vi "PH_VacuumControl.PC Write PSDB.vi"(0 "i ref in":refnum<vi>, 5 "error IO":errorcluster) -> (14 "i ref out":refnum<vi>, 19 "error out":errorcluster)   [LabVIEW 2014, in "PH_VacuumControl.lvlib"]
doc: "This is the proc case which writes data to the PHELIX shot data base."
uses:
  PH_VacuumControl.lvlib
  PH_PSDBWriter/PH_PSDBWriter.2D dataset.ctl
  User/Eisenbarth/psdb_lv/PSDB_AxisDescription.ctl
  PH_PSDBWriter/PH_PSDBWriter.Numeric dataset.ctl
  PH_PSDBWriter/PH_PSDBWriter.lvlib
  User/Eisenbarth/psdb_lv/PSDB.lvlib
  PH_Common/PH_Common.lvlib
panel:
  in  "2D data":T1
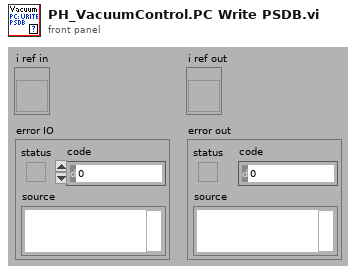
[diagram p1: front panel]
types:
  T1 = typedef "PH_PSDBWriter.lvlib/PH_PSDBWriter.2D dataset.ctl" = cluster{"name":string, "data":dbl[][], "axis description":T2}
  T2 = typedef "PSDB.lvlib/PSDB_AxisDescription.ctl" = cluster{"x axis label":string, "y axis label":string, "x axis unit":string, "y axis unit":string}
  T3 = typedef "PH_PSDBWriter.lvlib/PH_PSDBWriter.Numeric dataset.ctl" = cluster{"name":string, "data":dbl, "unit":string}
  T4 = typedef "PH_VacuumControl.lvlib/PH_VacuumControl.i attribute.ctl" = cluster{"GUI Refs":cluster{"Exit":refnum<vi>, "Set Unit":refnum<vi>, "Device found":refnum<vi>, "Busy":refnum<vi>, "State":refnum<vi>, "Delete":refnum<vi>, "Channels":refnum<vi>, "Channel Name":refnum<vi>, "Trend":refnum<vi>, "Logarithmic":refnum<vi>, "Limit reached":refnum<vi>, "Channel Name 1 MT":refnum<vi>, "Channel Name 2 MT":refnum<vi>, "Trend MT":refnum<vi>, "Logarithmic MT":refnum<vi>, "Limit reached MT":refnum<vi>}, "Device found":bool, "Busy":bool, "Selected Unit":i32, "Channels [mbar]":T5, "Channel Names":cluster{"Channel 1":string, "Channel 2":string, "Channel 3":string, "Channel 4":string, "Channel 5":string, "Channel 6":string}, "Status":T6, "AGCxxx VISA Cluster":T7, "Instr Firmware Revision":string, "Service IDs Pressure":cluster{"Channel 1":i32, "Channel 2":i32, "Channel 3":i32, "Channel 4":i32, "Channel 5":i32, "Channel 6":i32}, "Service IDs Limits":cluster{"Channel 1":i32, "Channel 2":i32, "Channel 3":i32, "Channel 4":i32, "Channel 5":i32, "Channel 6":i32}, "Trend":cluster{"Start Point":timestamp, "Pressures [mbar] Channel 1":dbl[], "Pressures [mbar] Channel 2":dbl[], "Pressures [mbar] Channel 3":dbl[], "Pressures [mbar] Channel 4":dbl[], "Pressures [mbar] Channel 5":dbl[], "Pressures [mbar] Channel 6":dbl[], "Timebase [s]":i32[], "Trend Channel":u16, "Start Fit":dbl, "Trend Channel 1 MT":u16, "Trend Channel 2 MT":u16, "Start or continue Fit MT":dbl, "Continue or start Fit MT":dbl, "Datasets strored":i32, "Dataarray Size":i32}, "Running":bool}
  T5 = typedef "PH_VacuumControl.lvlib/PH_VacuumControl.Channels.ctl" = cluster{"Channel 1":dbl, "Channel 2":dbl, "Channel 3":dbl, "Channel 4":dbl, "Channel 5":dbl, "Channel 6":dbl, "Name Channel 1":string, "Name Channel 2":string, "Name Channel 3":string, "Name Channel 4":string, "Name Channel 5":string, "Name Channel 6":string, "Upper Limit":dbl, "Upper Limit 2":dbl, "Upper Limit 3":dbl, "Upper Limit 4":dbl, "Upper Limit 5":dbl, "Upper Limit 6":dbl}
  T6 = typedef "PH_StatusHandler.lvlib/PH_StatusHandler.Status.ctl" = i16
  T7 = typedef "AGCxxx - Driver.lvlib/AGCxxx VISA Control.ctl" = cluster{"VISA resource name":refnum<visa-resource-name>, "VISA Timeout Value (1000 ms)":u32, "Lock Timeout (1000 ms)":u32, "MAX Channel (6)":i32}
  T8 = typedef "PH_PSDBWriter.lvlib/PH_PSDBWriter.String dataset.ctl" = cluster{"name":string, "data":string, "unit":string}
  T9 = typedef "PH_PSDBWriter.lvlib/PH_PSDBWriter.PSDB Dataset.ctl" = cluster{"Version":i32, "2D data Input":T1[], "Boolean Input":T10[], "Image Input":T11[], "Numeric Input":T3[], "String Input":T8[]}
  T10 = typedef "PH_PSDBWriter.lvlib/PH_PSDBWriter.Boolean dataset.ctl" = cluster{"name":string, "data":bool, "unit":string}
  T11 = typedef "PH_PSDBWriter.lvlib/PH_PSDBWriter.Image dataset.ctl" = cluster{"name":string, "data":T12, "unit":string}
  T12 = typedef "IMAQ Image.ctl" = refnum<image>
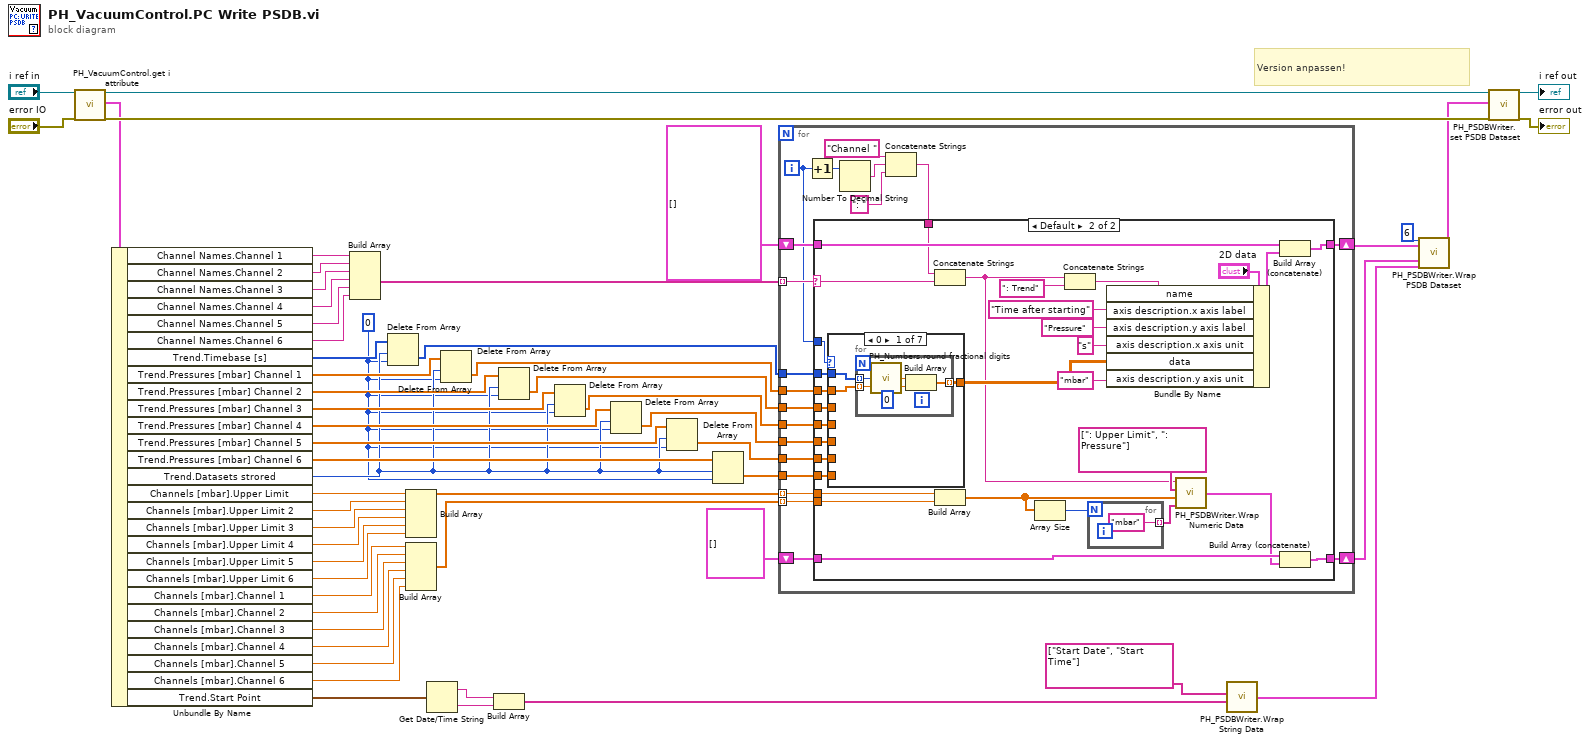
[diagram p0: block diagram]
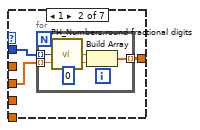
[diagram p3: hidden frame]
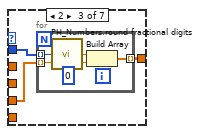
[diagram p4: hidden frame]
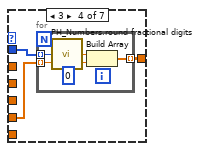
[diagram p5: hidden frame]
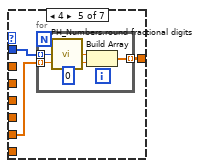
[diagram p6: hidden frame]
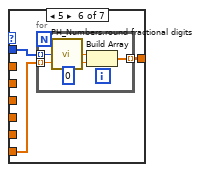
[diagram p7: hidden frame]
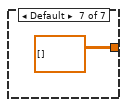
[diagram p8: hidden frame]
diagram:
  w14 = 0 ("index")
  # "Version anpassen!"
  n1 = call "PH_VacuumControl.get i attribute.vi"("i ref in"="i ref in", "error in (no error)"="error IO") -> ("i ref out"=w12:refnum<vi>, "i attribute"=w39:T4, "error out"=w54:errorcluster)  [unwired: 15 in]
  n2 = Unbundle By Name(w39) -> ("Channel Names.Channel 1"=w53:string, "Channel Names.Channel 2"=w52:string, "Channel Names.Channel 3"=w51:string, "Channel Names.Channel 4"=w50:string, "Channel Names.Channel 5"=w49:string, "Channel Names.Channel 6"=w48:string, "Trend.Timebase [s]"=w26:i32[], "Trend.Pressures [mbar] Channel 1"=w25:dbl[], "Trend.Pressures [mbar] Channel 2"=w24:dbl[], "Trend.Pressures [mbar] Channel 3"=w22:dbl[], "Trend.Pressures [mbar] Channel 4"=w21:dbl[], "Trend.Pressures [mbar] Channel 5"=w20:dbl[], "Trend.Pressures [mbar] Channel 6"=w19:dbl[], "Trend.Datasets strored"=w16:i32, "Channels [mbar].Upper Limit"=w47:dbl, "Channels [mbar].Upper Limit 2"=w46:dbl, "Channels [mbar].Upper Limit 3"=w45:dbl, "Channels [mbar].Upper Limit 4"=w44:dbl, "Channels [mbar].Upper Limit 5"=w43:dbl, "Channels [mbar].Upper Limit 6"=w42:dbl, "Channels [mbar].Channel 1"=w33:dbl, "Channels [mbar].Channel 2"=w32:dbl, "Channels [mbar].Channel 3"=w31:dbl, "Channels [mbar].Channel 4"=w30:dbl, "Channels [mbar].Channel 5"=w29:dbl, "Channels [mbar].Channel 6"=w28:dbl, "Trend.Start Point"=w34:timestamp)
  n3 = Build Array(w53, w52, w51, w50, w49, w48) -> (w40:string[])
  n4 = Delete From Array(array=w26, length=w16, index=w14) -> (deleted portion=w15:i32[])  [unwired: 1 out]
  n5 = Build Array(w47, w46, w45, w44, w43, w42) -> (w41:dbl[])
  n6 = Build Array(w33, w32, w31, w30, w29, w28) -> (w27:dbl[])
  n7 = Get Date/Time String(seconds (now)=w34) -> (date string=w36:string, time string=w35:string)  [unwired: 2 in]
  n8 = Delete From Array(array=w25, length=w16, index=w14) -> (deleted portion=w23:dbl[])  [unwired: 1 out]
  n9 = Build Array(w36, w35) -> (w6:string[])
  n10 = Delete From Array(array=w24, length=w16, index=w14) -> (deleted portion=w1:dbl[])  [unwired: 1 out]
  n11 = Delete From Array(array=w22, length=w16, index=w14) -> (deleted portion=w2:dbl[])  [unwired: 1 out]
  n12 = Delete From Array(array=w21, length=w16, index=w14) -> (deleted portion=w3:dbl[])  [unwired: 1 out]
  n13 = Delete From Array(array=w20, length=w16, index=w14) -> (deleted portion=w17:dbl[])  [unwired: 1 out]
  n14 = Delete From Array(array=w19, length=w16, index=w14) -> (deleted portion=w18:dbl[])  [unwired: 1 out]
  n15 = for {
    tunnel: w41 -> [w76] mode=indexing
    shift-right: [w75] -> w7
    shift-left: T1[] [] ("Vacuum Control PSDB 2D Data") -> [w74]
    tunnel: w40 -> [w73] mode=indexing
    shift-right: [w72] -> w8
    shift-left: T3[] [] -> [w71]
    tunnel: w15 -> [w65]
    tunnel: w23 -> [w64]
    tunnel: w1 -> [w63]
    tunnel: w2 -> [w62]
    tunnel: w3 -> [w61]
    tunnel: w17 -> [w60]
    tunnel: w18 -> [w59]
    tunnel: w27 -> [w57] mode=indexing
    i -> [w58]
    n16 = Increment(x=w58) -> (x+1=w67:i32)
    n17 = Number To Decimal String(number=w67) -> (decimal integer string=w68:string)  [unwired: 1 in]
    n18 = Concatenate Strings("Channel " ("string"), w68, ": " ("string")) -> (w66:string)
    n19 = case shown="Default" w73 {
      selector: w73 -> [_ w84]
      tunnel: w76 -> [_ w87]
      tunnel: [w78 w109] -> w75
      tunnel: w74 -> [w78 w108]
      tunnel: [w77 w106] -> w72
      tunnel: w71 -> [w77 w105]
      tunnel: w66 -> [_ w85]
      tunnel: w65 -> [_ w97]
      tunnel: w64 -> [_ w96]
      tunnel: w63 -> [_ w93]
      tunnel: w62 -> [_ w92]
      tunnel: w61 -> [_ w91]
      tunnel: w60 -> [_ w90]
      tunnel: w59 -> [_ w89]
      tunnel: w58 -> [_ w94]
      tunnel: w57 -> [_ w88]
      frame "", "N/A" {
      }
      frame Default {
        n20 = case shown="0" w94 {
          tunnel: [w113 w121 w129 w137 w145 w153 dbl[][] []] -> w98
          tunnel: w97 -> [w112 w120 w128 w136 w144 w152 _]
          tunnel: w96 -> [w111 _ _ _ _ _ _]
          tunnel: w93 -> [_ w119 _ _ _ _ _]
          tunnel: w92 -> [_ _ w127 _ _ _ _]
          tunnel: w91 -> [_ _ _ w135 _ _ _]
          tunnel: w90 -> [_ _ _ _ w143 _ _]
          tunnel: w89 -> [_ _ _ _ _ w151 _]
          frame 0 {
            n21 = for {
              tunnel: w112 -> [w117] mode=indexing
              tunnel: w111 -> [w114] mode=indexing
              tunnel: [w118] -> w113 mode=indexing
              n22 = call "PH_Numbers.round fractional digits.vi"("Input"=w117, "Position (1)"=i16 0) -> ("round Output"=w116:dbl)
              n23 = Build Array(w116, w114) -> (w118:dbl[])
            }
          }
          frame 1 {
            n24 = for {
              tunnel: w120 -> [w125] mode=indexing
              tunnel: w119 -> [w122] mode=indexing
              tunnel: [w126] -> w121 mode=indexing
              n25 = call "PH_Numbers.round fractional digits.vi"("Input"=w125, "Position (1)"=i16 0) -> ("round Output"=w124:dbl)
              n26 = Build Array(w124, w122) -> (w126:dbl[])
            }
          }
          frame 2 {
            n27 = for {
              tunnel: w128 -> [w133] mode=indexing
              tunnel: w127 -> [w130] mode=indexing
              tunnel: [w134] -> w129 mode=indexing
              n28 = call "PH_Numbers.round fractional digits.vi"("Input"=w133, "Position (1)"=i16 0) -> ("round Output"=w132:dbl)
              n29 = Build Array(w132, w130) -> (w134:dbl[])
            }
          }
          frame 3 {
            n30 = for {
              tunnel: w136 -> [w141] mode=indexing
              tunnel: w135 -> [w138] mode=indexing
              tunnel: [w142] -> w137 mode=indexing
              n31 = call "PH_Numbers.round fractional digits.vi"("Input"=w141, "Position (1)"=i16 0) -> ("round Output"=w140:dbl)
              n32 = Build Array(w140, w138) -> (w142:dbl[])
            }
          }
          frame 4 {
            n33 = for {
              tunnel: w144 -> [w149] mode=indexing
              tunnel: w143 -> [w146] mode=indexing
              tunnel: [w150] -> w145 mode=indexing
              n34 = call "PH_Numbers.round fractional digits.vi"("Input"=w149, "Position (1)"=i16 0) -> ("round Output"=w148:dbl)
              n35 = Build Array(w148, w146) -> (w150:dbl[])
            }
          }
          frame 5 {
            n36 = for {
              tunnel: w152 -> [w157] mode=indexing
              tunnel: w151 -> [w154] mode=indexing
              tunnel: [w158] -> w153 mode=indexing
              n37 = call "PH_Numbers.round fractional digits.vi"("Input"=w157, "Position (1)"=i16 0) -> ("round Output"=w156:dbl)
              n38 = Build Array(w156, w154) -> (w158:dbl[])
            }
          }
          frame Default {
          }
        }
        n39 = Concatenate Strings(w85, w84) -> (w79:string)
        n40 = Build Array(w87, w88) -> (w82:dbl[])
        n41 = Array Size(array=w82) -> (size(s)=w83:i32)
        n42 = Concatenate Strings(w79, ": Trend" ("string")) -> (w102:string)
        n43 = for {
          N: w83 -> [_]
          tunnel: ["mbar" ("unit")] -> w81 mode=indexing
        }
        n44 = Bundle By Name(cluster="2D data", "name"=w102, "axis description.x axis label"="Time after starting", "axis description.y axis label"="Pressure", "axis description.x axis unit"="s", "data"=w98, "axis description.y axis unit"="mbar" ("unit")) -> (w103:T1)
        n45 = call "PH_PSDBWriter.Wrap Numeric Data.vi"("Unit Array"=w81, "Data Array"=w82, "Name Array"=string[] [": Upper Limit", ": Pressure"], "Name Prefix"=w79) -> ("PSDB Numeric Data Array"=w80:T3[])
        n46 = Build Array (concatenate)(w108, w103) -> (w109:T1[])
        n47 = Build Array (concatenate)(w105, w80) -> (w106:T3[])
      }
    }
  }
  n48 = call "PH_PSDBWriter.Wrap String Data.vi"("Data Array"=w6, "Name Array"=string[] ["Start Date", "Start Time"]) -> ("PSDB String Data Array"=w4:T8[])  [unwired: 2 in]
  n49 = call "PH_PSDBWriter.Wrap PSDB Dataset.vi"("Version"=6, "2D data Input"=w7, "Numeric Input"=w8, "String Input"=w4) -> ("PSDB Dataset"=w10:T9)  [unwired: 15 in]
  n50 = call "PH_PSDBWriter.set PSDB Dataset.vi"("VI in"=w12, "PSDB Dataset"=w10, "error in (no error)"=w54) -> ("VI out"=→"i ref out":refnum<vi>, "error out"=→"error out":errorcluster)  [unwired: 15 in]
